vi "Write Access Index.vi"(8 "error in (no error)":errorcluster, 10 "Access Index":u32, 11 "Var_Index in":refnum<class "Bus_Index.lvclass">) -> (0 "error out":errorcluster, 3 "Var_Index out":refnum<class "Bus_Index.lvclass">)   [LabVIEW 2021, in "Bus_Index.lvclass"]
uses:
  Bus_Index.lvclass
  Bus_Index.lvclass/Bus_Index.ctl
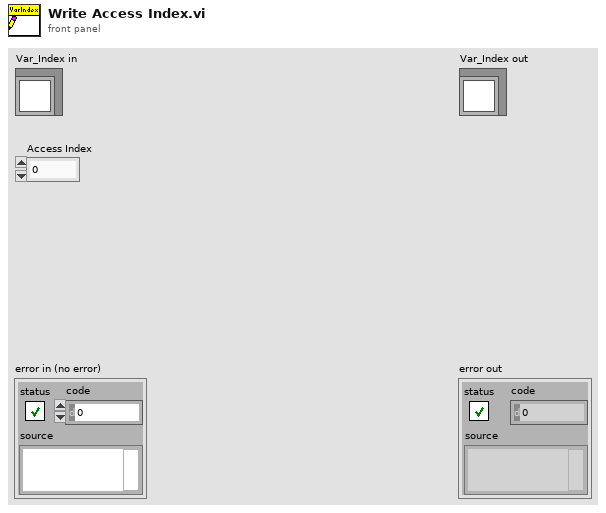
[diagram p1: front panel]
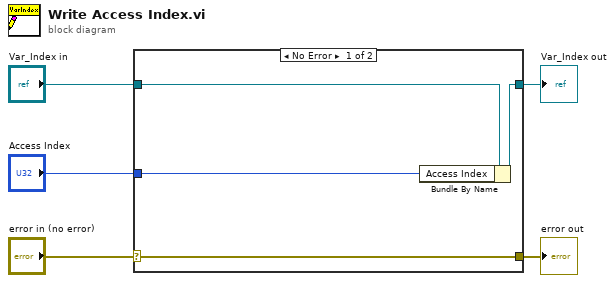
[diagram p0: block diagram]
diagram:
  n1 = case shown="No Error" "error in (no error)" {
    selector: "error in (no error)" -> [w9 w10]
    tunnel: [w9 w10] -> w4
    tunnel: [w7 w11] -> w2
    tunnel: "Var_Index in" -> [w8 w11]
    tunnel: "Access Index" -> [w6 _]
    frame No Error {
      n2 = Bundle By Name(cluster=w8, "Access Index"=w6) -> (w7:refnum<class "Bus_Index.lvclass">)
    }
    frame Error {
    }
  }
  "error out" <- w4
  "Var_Index out" <- w2
